vi "closeDocument.vi"(8 "error in (no error)":errorcluster, 11 "MS-Word in":refnum<class "MS-Word.lvclass">) -> (0 "error out":errorcluster, 3 "MS-Word out":refnum<class "MS-Word.lvclass">)   [LabVIEW 2017, in "LabVIEW NPOI.lvlib" / "MS-Word.lvclass"]
doc: "Protected dynamic dispatch method to close the <b>Document</b>."
uses:
  MS-Word.lvclass
  MS-Word.lvclass/MS-Word.ctl
  xwpfDocument/xwpfDocument.lvclass
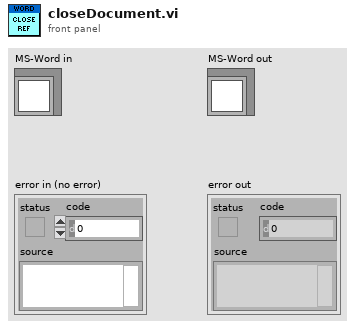
[diagram p1: front panel]
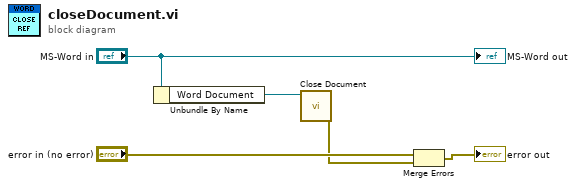
[diagram p0: block diagram]
diagram:
  n1 = Unbundle By Name("MS-Word in") -> ("Word Document"=w4:refnum<class "xwpfDocument.lvclass">)
  n2 = call "Close Document.vi"("xwpfDocument in"=w4) -> ("error out"=w1:errorcluster)  [unwired: 9 in, 1 out]
  n3 = Merge Errors("error in (no error)", w1) -> (→"error out":errorcluster)
  "MS-Word out" <- "MS-Word in"
